vi "Test Char Array.vi"() -> ()   [LabVIEW 2020, in "Terminal.lvlib" / "TermBuffer.lvclass"]
uses:
  TermBuffer.lvclass
  Term Char.ctl
  Terminal.lvlib
panel:
  out "TermChars":T1[][](array[typedef])
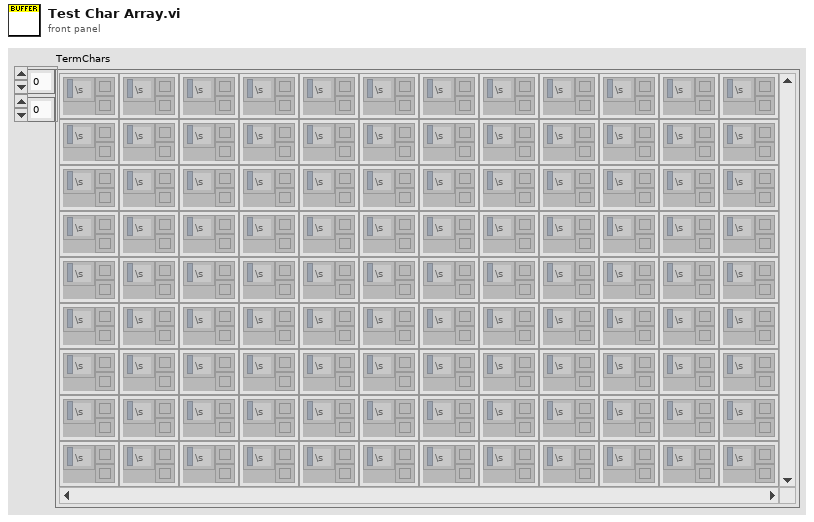
[diagram p1: front panel]
types:
  T1 = typedef "Terminal.lvlib/Term Char.ctl" = cluster{"Char":string, "FG":u32, "BG":u32}
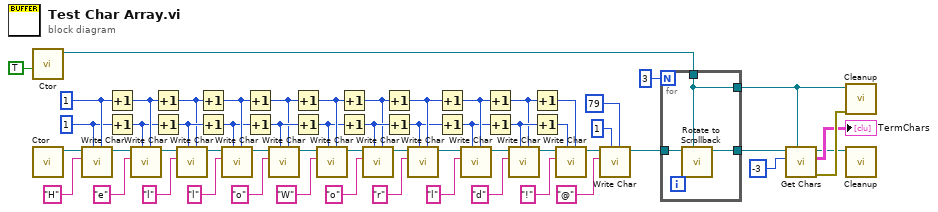
[diagram p0: block diagram]
diagram:
  w55 = 1 ("Col")
  w54 = 1 ("Row")
  n1 = call "Ctor.vi"("Is Scrollback? (F)"=TRUE) -> ("TermBuffer out"=w7:refnum<class "TermBuffer.lvclass">)  [unwired: 9 in, 1 out]
  n2 = call "Ctor.vi"() -> ("TermBuffer out"=w57:refnum<class "TermBuffer.lvclass">)  [unwired: 10 in, 1 out]
  n3 = call "Write Char.vi"("Col"=w55, "Row"=w54, "Char"="H", "TermBuffer in"=w57) -> ("TermBuffer out"=w53:refnum<class "TermBuffer.lvclass">)  [unwired: 6 in, 1 out]
  n4 = Increment(x=w55) -> (x+1=w40:i32)
  n5 = Increment(x=w54) -> (x+1=w39:i32)
  n6 = call "Write Char.vi"("Col"=w40, "Row"=w39, "Char"="e", "TermBuffer in"=w53) -> ("TermBuffer out"=w14:refnum<class "TermBuffer.lvclass">)  [unwired: 6 in, 1 out]
  n7 = Increment(x=w40) -> (x+1=w37:i32)
  n8 = Increment(x=w39) -> (x+1=w38:i32)
  n9 = call "Write Char.vi"("Col"=w37, "Row"=w38, "Char"="l", "TermBuffer in"=w14) -> ("TermBuffer out"=w15:refnum<class "TermBuffer.lvclass">)  [unwired: 6 in, 1 out]
  n10 = Increment(x=w37) -> (x+1=w36:i32)
  n11 = Increment(x=w38) -> (x+1=w35:i32)
  n12 = call "Write Char.vi"("Col"=w36, "Row"=w35, "Char"="l", "TermBuffer in"=w15) -> ("TermBuffer out"=w16:refnum<class "TermBuffer.lvclass">)  [unwired: 6 in, 1 out]
  n13 = Increment(x=w36) -> (x+1=w33:i32)
  n14 = Increment(x=w35) -> (x+1=w34:i32)
  n15 = call "Write Char.vi"("Col"=w33, "Row"=w34, "Char"="o", "TermBuffer in"=w16) -> ("TermBuffer out"=w17:refnum<class "TermBuffer.lvclass">)  [unwired: 6 in, 1 out]
  n16 = Increment(x=w33) -> (x+1=w32:i32)
  n17 = Increment(x=w34) -> (x+1=w31:i32)
  n18 = call "Write Char.vi"("Col"=w32, "Row"=w31, "Char"="W", "TermBuffer in"=w17) -> ("TermBuffer out"=w18:refnum<class "TermBuffer.lvclass">)  [unwired: 6 in, 1 out]
  n19 = Increment(x=w32) -> (x+1=w29:i32)
  n20 = Increment(x=w31) -> (x+1=w30:i32)
  n21 = call "Write Char.vi"("Col"=w29, "Row"=w30, "Char"="o", "TermBuffer in"=w18) -> ("TermBuffer out"=w19:refnum<class "TermBuffer.lvclass">)  [unwired: 6 in, 1 out]
  n22 = Increment(x=w29) -> (x+1=w28:i32)
  n23 = Increment(x=w30) -> (x+1=w27:i32)
  n24 = call "Write Char.vi"("Col"=w28, "Row"=w27, "Char"="r", "TermBuffer in"=w19) -> ("TermBuffer out"=w20:refnum<class "TermBuffer.lvclass">)  [unwired: 6 in, 1 out]
  n25 = Increment(x=w28) -> (x+1=w26:i32)
  n26 = Increment(x=w27) -> (x+1=w25:i32)
  n27 = call "Write Char.vi"("Col"=w26, "Row"=w25, "Char"="l", "TermBuffer in"=w20) -> ("TermBuffer out"=w21:refnum<class "TermBuffer.lvclass">)  [unwired: 6 in, 1 out]
  n28 = Increment(x=w26) -> (x+1=w23:i32)
  n29 = Increment(x=w25) -> (x+1=w24:i32)
  n30 = call "Write Char.vi"("Col"=w23, "Row"=w24, "Char"="d", "TermBuffer in"=w21) -> ("TermBuffer out"=w22:refnum<class "TermBuffer.lvclass">)  [unwired: 6 in, 1 out]
  n31 = Increment(x=w23) -> (x+1=w42:i32)
  n32 = Increment(x=w24) -> (x+1=w41:i32)
  n33 = call "Write Char.vi"("Col"=w42, "Row"=w41, "Char"="!", "TermBuffer in"=w22) -> ("TermBuffer out"=w13:refnum<class "TermBuffer.lvclass">)  [unwired: 6 in, 1 out]
  n34 = call "Write Char.vi"("Col"=79 ("Row"), "Row"=1, "Char"="@", "TermBuffer in"=w13) -> ("TermBuffer out"=w9:refnum<class "TermBuffer.lvclass">)  [unwired: 6 in, 1 out]
  n35 = for {
    N: 3 -> [_]
    tunnel: w9 -> [w61]
    tunnel: w7 -> [w60]
    tunnel: [w60] -> w2
    tunnel: [w59] -> w5
    n36 = call "Rotate to Scrollback.vi"("Scrollback"=w60, "TermBuffer in"=w61) -> ("TermBuffer out"=w59:refnum<class "TermBuffer.lvclass">)  [unwired: 8 in, 1 out]
  }
  n37 = call "Get Chars.vi"("Scrollback"=w2, "Start (Beginning)"=-3, "TermBuffer in"=w5) -> ("error out"=w58:errorcluster, "TermChars"=→"TermChars":T1[][], "TermBuffer out"=w1:refnum<class "TermBuffer.lvclass">)  [unwired: 6 in]
  n38 = call "Cleanup.vi"("error in (no error)"=w58, "TermBuffer in"=w2) -> ()  [unwired: 9 in, 1 out]
  n39 = call "Cleanup.vi"("TermBuffer in"=w1) -> ()  [unwired: 10 in, 1 out]
